vi "Query.vi"(6 "error":errorcluster, 8 "Quantity":string(combo)="Temperature[C]", 9 "VISA resource name":refnum<visa-resource-name>="COM1") -> (0 "error out":errorcluster, 2 "Value":dbl=39.0 format="%_4f", 3 "VISA resource name out":refnum<visa-resource-name>="COM1", 5 "Response":string="temp. CG 39 d  \r\n")   [LabVIEW 2023, in "BigSkyControl.lvlib"]
uses:
  BigSkyControl.lvlib
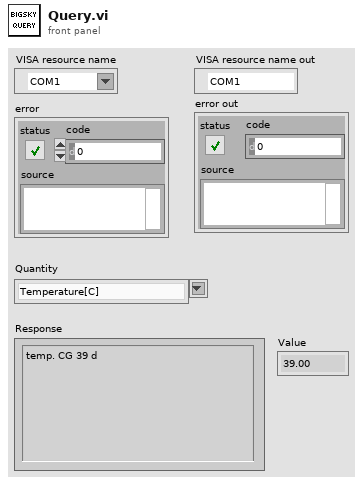
[diagram p1: front panel]
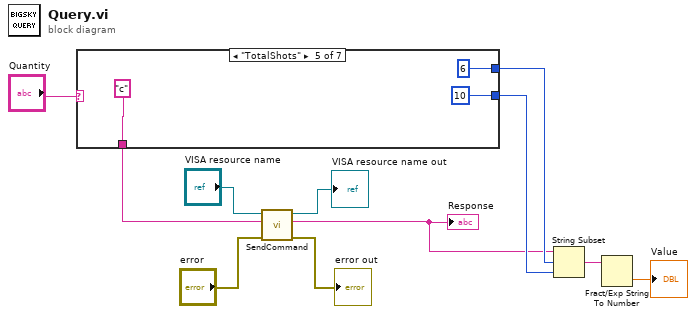
[diagram p0: block diagram]
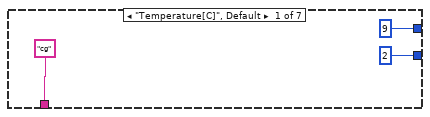
[diagram p2: hidden frame]
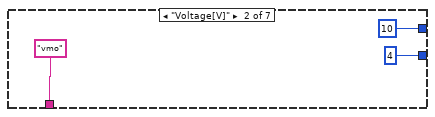
[diagram p3: hidden frame]
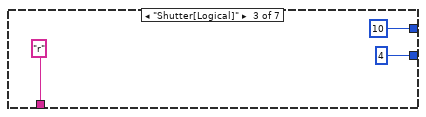
[diagram p4: hidden frame]
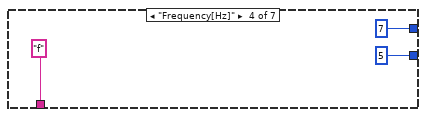
[diagram p5: hidden frame]
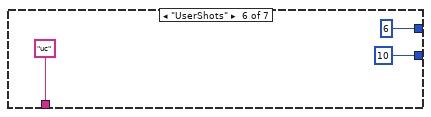
[diagram p6: hidden frame]
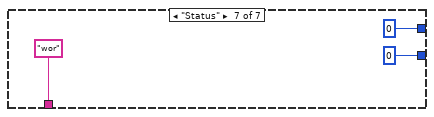
[diagram p7: hidden frame]
diagram:
  n1 = case shown="\"TotalShots\"" "Quantity" {
    tunnel: ["cg" ("write buffer") "vmo" ("write buffer") "r" ("write buffer") "f" ("write buffer") "c" ("write buffer") "uc" ("write buffer") "wor" ("write buffer")] -> w5
    tunnel: [9 ("offset (0)") 10 ("offset (0)") 10 ("offset (0)") 7 ("offset (0)") 6 ("offset (0)") 6 ("offset (0)") 0 ("offset (0)")] -> w10
    tunnel: [2 ("length (rest)") 4 ("length (rest)") 4 ("length (rest)") 5 ("length (rest)") 10 ("length (rest)") 10 ("length (rest)") 0 ("length (rest)")] -> w9
    frame "Temperature[C]", Default {
    }
    frame "Voltage[V]" {
    }
    frame "Shutter[Logical]" {
    }
    frame "Frequency[Hz]" {
    }
    frame "TotalShots" {
    }
    frame "UserShots" {
    }
    frame "Status" {
    }
  }
  n2 = call "SendCommand.vi"("error"="error", "write buffer (don't include >\\r\\n)"=w5, "VISA resource name"="VISA resource name") -> ("error out"=→"error out":errorcluster, "Response"=w2:string, "VISA resource name out"=→"VISA resource name out":refnum<visa-resource-name>)  [unwired: 6 in]
  "Response" <- w2
  n3 = String Subset(string=w2, offset (0)=w10, length (rest)=w9) -> (substring=w11:string)
  n4 = Fract/Exp String To Number(string=w11) -> (number=→"Value":dbl)  [unwired: 3 in, 1 out]
